vi "Setup Dialog.vi"(0 "State In":T3) -> (4 "State Out":T3, 8 "canceled?":bool)   [LabVIEW 2020, in "KTable.xctl"]
uses:
  KTable.xctl
  State.ctl
  ColumnSpec.ctl
  ColumnType.ctl
  Table Properties.ctl
  Events.ctl
  Event Data.ctl
  Event Type.ctl
  KListbox/KListbox.xctl
  Buttons/KCheckmarkBoolean 2.ctl
panel:
  in  "Show row headers":T1
  in  "Max rows":i32
  in  "User can add/delete rows":T1
  in  "Vertical scrollbar":T1
  out "redisplay":bool
  in  "Tab (top)":enum32{"Page 2"}(tab)
  in  "Name":string
  in  "Type":T2(ring)
  in  "Width":i32
  in  "Position":enum16{"Left", "Center", "Right"}(ring)
  in  "Locked":T1
  in  "Delete Button":bool
  in  "Add Button":bool
  out "cancel signal":bool
  in  "Cancel Button":bool
  in  "OK Button":bool
  in  "Tab (bottom)":T8(tab)
  out "EnumValues":string
  in  "EnumPath":path
  in  "Hide NaN":T1
  in  "False":string
  in  "True":string
  in  "Strings":cluster{"Row":i32, "Items":string[]}(xcontrol)
  in  "Columns":i32(listbox)
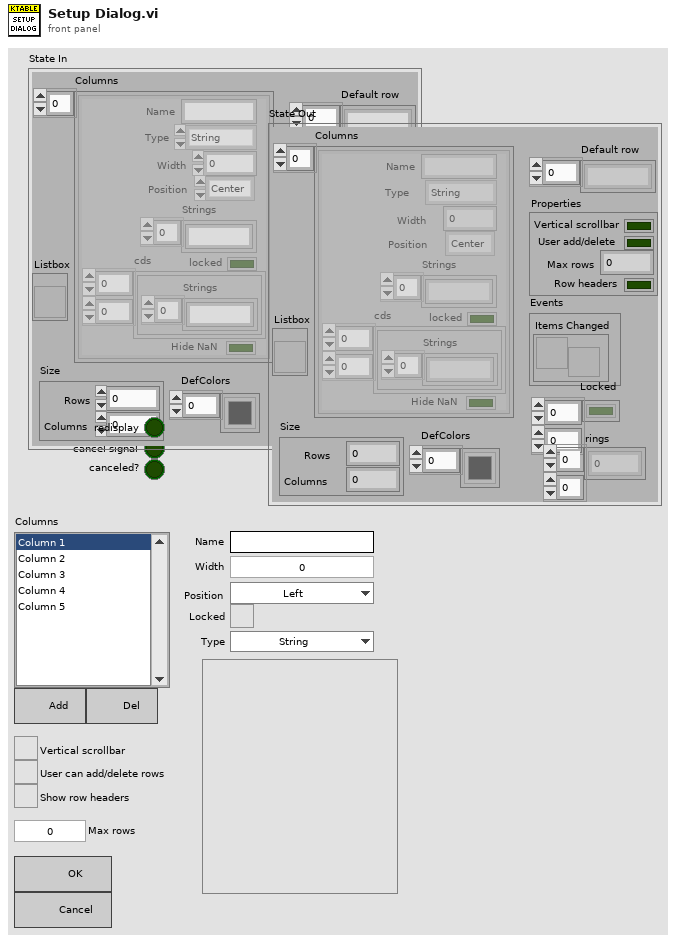
[diagram p1: front panel]
types:
  T1 = typedef "KCheckmarkBoolean 2.ctl" = bool
  T2 = enum16{"String", "Enum", "Int", "Double", "Boolean", "Ring", "Formula", "Color"}
  T3 = typedef "KTable.xctl/State.ctl" = cluster{"Columns":T4[], "Listbox":refnum<vi>, "Default row":string[], "Properties":T6, "Events":T7, "Locked":bool[][], "Size":cluster{"Rows":i32, "Columns":i32}, "rings":i32[][], "DefColors":u32[]}
  T4 = typedef "KTable.xctl/ColumnSpec.ctl" = cluster{"Name":string, "Type":T5, "Width":i32, "Strings":string[], "Position":enum16{"Left", "Center", "Right"}, "locked":bool, "cds":cluster{"Strings":string[]}[][], "Hide NaN":bool}
  T5 = typedef "KTable.xctl/ColumnType.ctl" = enum16{"String", "Enum", "Int", "Double", "Boolean", "Ring", "Formula", "Color"}
  T6 = typedef "KTable.xctl/Table Properties.ctl" = cluster{"Vertical scrollbar":bool, "User add/delete":bool, "Max rows":i32, "Row headers":bool}
  T7 = typedef "KTable.xctl/Events.ctl" = cluster{"Items Changed":refnum<user-event>}
  T8 = enum32{"String", "Enum", "Int", "Double", "Boolean", "Ring", "Formula", "Color"}
  T9 = enum32{"String", "Enum", "Int", "Double", "Boolean", "Ring", "Formula"}
  T10 = enum8{"Enabled", "Disabled", "Disabled and Grayed Out"}
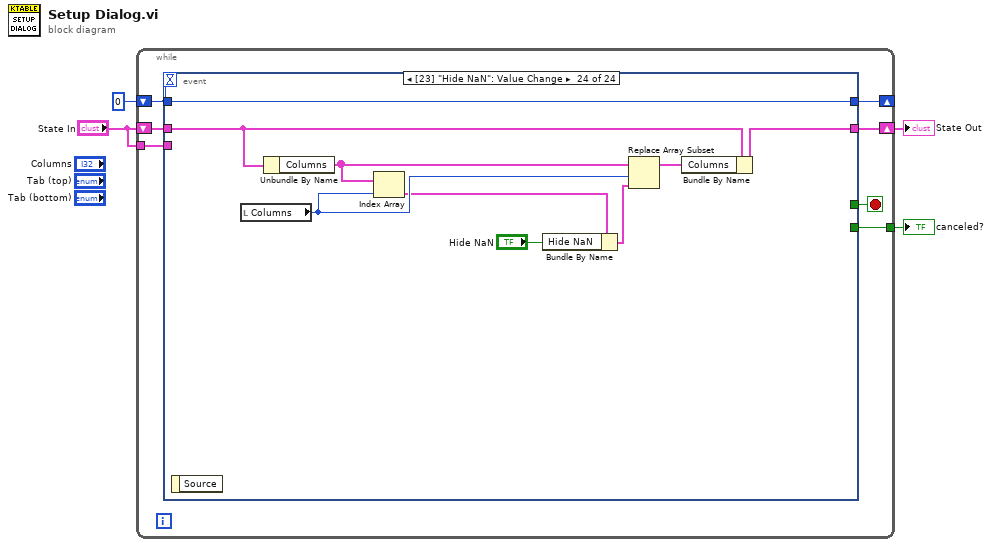
[diagram p0: block diagram]
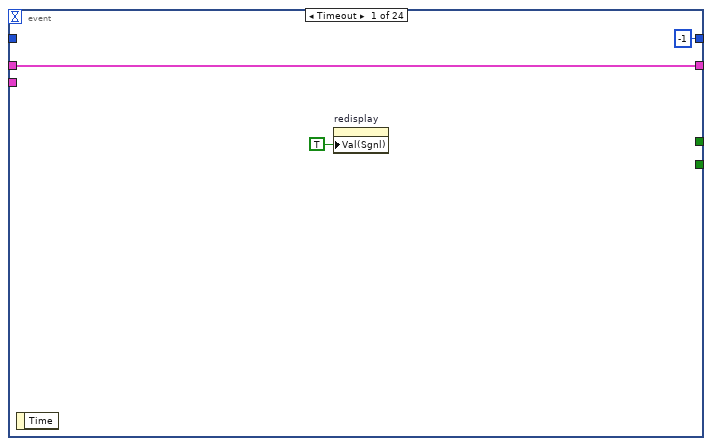
[diagram p2: hidden frame]
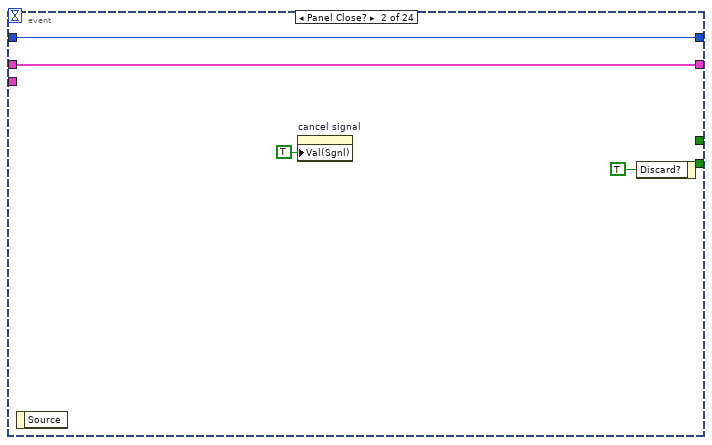
[diagram p3: hidden frame]
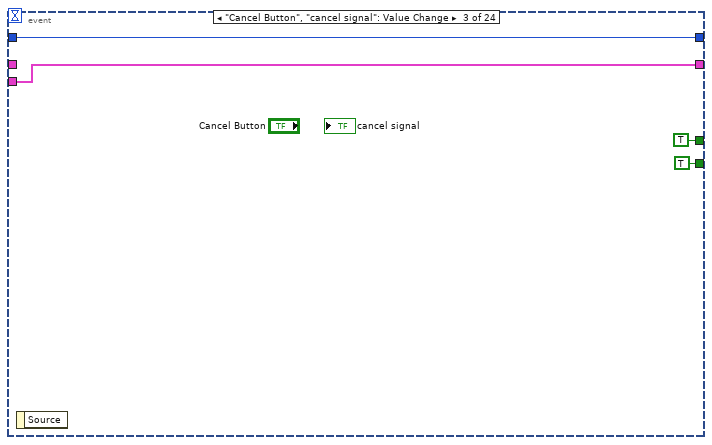
[diagram p4: hidden frame]
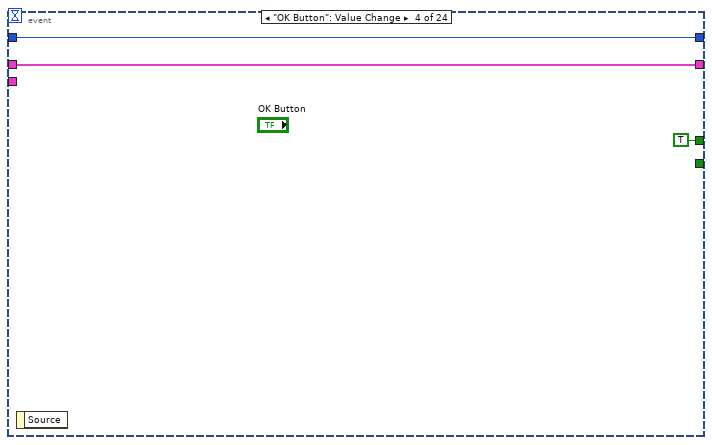
[diagram p5: hidden frame]
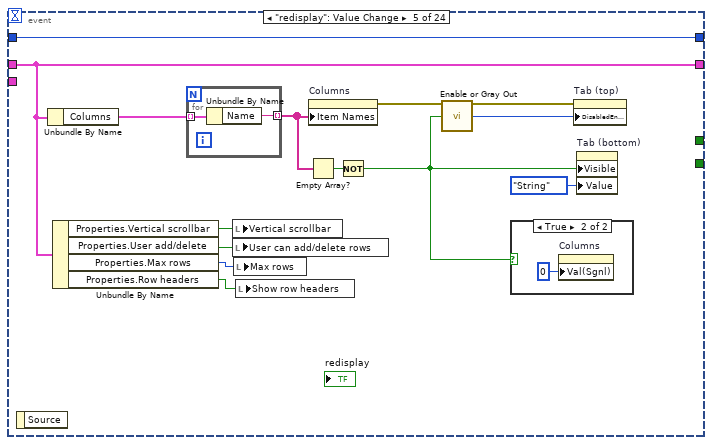
[diagram p6: hidden frame]
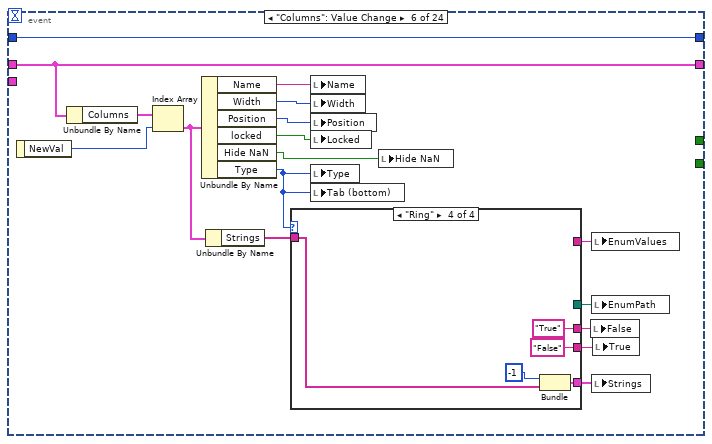
[diagram p8: hidden frame]
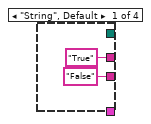
[diagram p9: hidden frame]
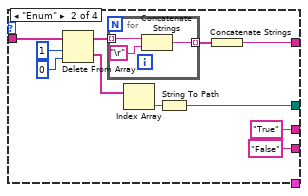
[diagram p10: hidden frame]
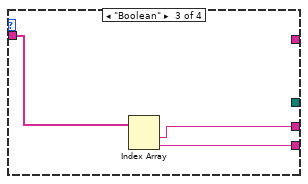
[diagram p11: hidden frame]
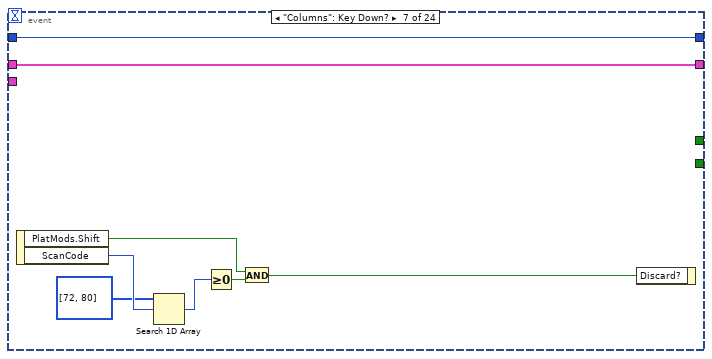
[diagram p12: hidden frame]
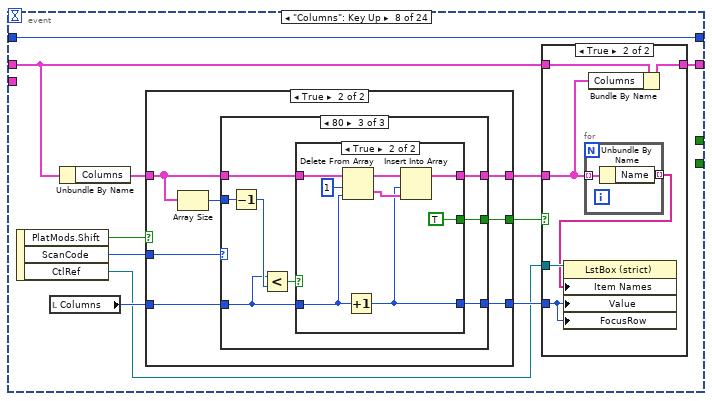
[diagram p13: hidden frame]
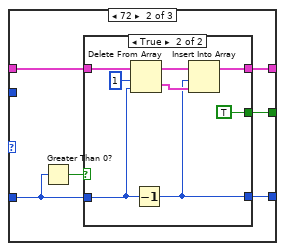
[diagram p17: hidden frame]
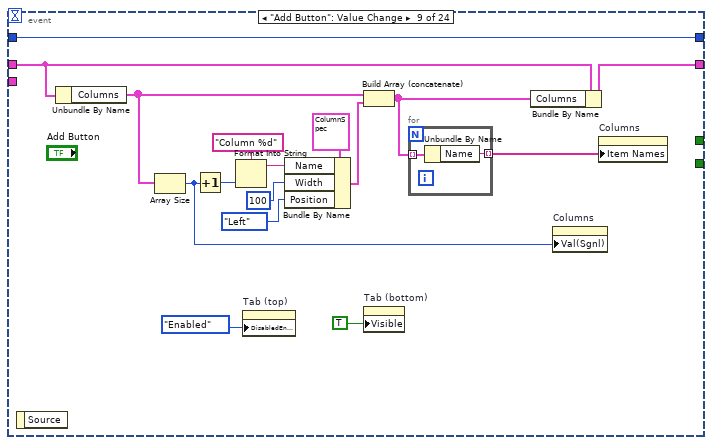
[diagram p20: hidden frame]
diagram:
  n1 = while {
    shift-right: [w10] -> _
    shift-left: 0 -> [w11]
    shift-right: [w7] -> w1
    shift-left: "State In" -> [w8]
    tunnel: "State In" -> [w6]
    tunnel: [w5] -> w2
    stop <- w9 stop-if-true
    n2 = event shown="[23] \"Hide NaN\": Value Change" {
      selector: _ -> [_ _ _ _ _ _ _ _ _ _ _ _ _ _ _ _ _ _ _ _ _ _ _ _]
      dyn-events: _ -> [_ _ _ _ _ _ _ _ _ _ _ _ _ _ _ _ _ _ _ _ _ _ _ _]
      timeout: w11 -> [_ _ _ _ _ _ _ _ _ _ _ _ _ _ _ _ _ _ _ _ _ _ _ _]
      tunnel: w11 -> [_ w18 w22 w25 w31 w58 w90 w101 w171 w180 w190 w194 w198 w202 w212 w225 w234 w243 w256 w274 w289 w301 w311 w320]
      tunnel: [-1 w18 w22 w25 w31 w58 w90 w101 w171 w180 w190 w194 w198 w202 w212 w225 w234 w243 w256 w274 w289 w301 w311 w320] -> w10
      tunnel: [_ _ TRUE TRUE _ _ _ _ _ _ _ _ _ _ _ _ _ _ _ _ _ _ _ _] -> w9
      tunnel: w8 -> [w13 w15 _ w23 w30 w57 w89 w96 w170 w179 w189 w193 w197 w201 w211 w224 w233 w242 w255 w273 w288 w300 w310 w319]
      tunnel: [w13 w15 w20 w23 w30 w57 w89 w95 w164 w176 w188 w192 w196 w200 w205 w219 w228 w237 w251 w268 w285 w297 w307 w316] -> w7
      tunnel: w6 -> [_ _ w20 _ _ _ _ _ _ _ _ _ _ _ _ _ _ _ _ _ _ _ _ _]
      tunnel: [_ _ TRUE _ _ _ _ _ _ _ _ _ _ _ _ _ _ _ _ _ _ _ _ _] -> w5
      event Timeout {
        n3 = event-data() -> ()  [unwired: 1 in, 1 out]
        n4 = property on="redisplay" class="Bool (strict)"("Val(Sgnl)"=TRUE ("Value (Signaling)")) -> ()  [unwired: 2 in, 2 out]
      }
      event Panel Close? {
        n5 = event-data() -> ()  [unwired: 1 in, 1 out]
        n6 = property on="cancel signal" class="Bool (strict)"("Val(Sgnl)"=TRUE ("Value (Signaling)")) -> ()  [unwired: 2 in, 2 out]
        n7 = event-data("Discard?"=TRUE) -> ()  [unwired: 1 in, 1 out]
      }
      event "Cancel Button", "cancel signal": Value Change {
        n8 = event-data() -> ()  [unwired: 1 in, 1 out]
      }
      event "OK Button": Value Change {
        n9 = event-data() -> ()  [unwired: 1 in, 1 out]
      }
      event "redisplay": Value Change {
        n10 = event-data() -> ()  [unwired: 1 in, 1 out]
        n11 = Unbundle By Name(w30) -> ("Columns"=w38:T4[])
        n12 = Unbundle By Name(w30) -> ("Properties.Vertical scrollbar"=w29:bool, "Properties.User add/delete"=w28:bool, "Properties.Max rows"=w27:i32, "Properties.Row headers"=w26:bool)
        n13 = for {
          tunnel: w38 -> [w41] mode=indexing
          tunnel: [w40] -> w37 mode=indexing
          n14 = Unbundle By Name(w41) -> ("Name"=w40:string)
        }
        n15 = local write "Vertical scrollbar"(w29) -> ()
        n16 = local write "User can add/delete rows"(w28) -> ()
        n17 = local write "Max rows"(w27) -> ()
        n18 = local write "Show row headers"(w26) -> ()
        n19 = Empty Array?(array=w37) -> (empty?=w35:bool)
        n20 = property on="Columns" class="LstBox (strict)"("Item Names"=w37) -> (error out=w36:errorcluster)  [unwired: 2 in, 1 out]
        n21 = Not(x=w35) -> (.not. x?=w33:bool)
        n22 = call "Enable or Gray Out.vi"("Boolean"=w33) -> ("Disabled"=w34:T10)
        n23 = case shown="True" w33 {
          frame False {
          }
          frame True {
            n24 = property on="Columns" class="LstBox (strict)"("Val(Sgnl)"=0 ("Value (Signaling)")) -> ()  [unwired: 2 in, 2 out]
          }
        }
        n25 = property on="Tab (top)" class="TabCtl (strict)"(error in=w36, "DisabledEnum"=w34) -> ()  [unwired: 1 in, 2 out]
        n26 = property on="Tab (bottom)" class="TabCtl (strict)"("Visible"=w33, "Value"=T9."String" ("Tab (bottom)")) -> ()  [unwired: 2 in, 2 out]
      }
      event "Columns": Value Change {
        n27 = event-data() -> ("NewVal"=w53:i32)  [unwired: 1 in]
        n28 = Unbundle By Name(w57) -> ("Columns"=w56:T4[])
        n29 = Index Array(array=w56, index=w53) -> (element=w51:T4)
        n30 = Unbundle By Name(w51) -> ("Name"=w55:string, "Width"=w54:i32, "Position"=w52:enum16{"Left", "Center", "Right"}, "locked"=w43:bool, "Hide NaN"=w42:bool, "Type"=w50:T5)
        n31 = Unbundle By Name(w51) -> ("Strings"=w49:string[])
        n32 = case shown="\"Ring\"" w50 {
          tunnel: w49 -> [_ w71 w77 w80]
          tunnel: [_ w67 _ _] -> w48
          tunnel: [_ w65 _ _] -> w47
          tunnel: ["True" ("String") "True" ("String") w76 "True" ("String")] -> w46
          tunnel: ["False" ("String") "False" ("String") w75 "False" ("String")] -> w45
          tunnel: [_ _ _ w78] -> w44
          frame "String", Default {
          }
          frame "Enum" {
            n33 = Delete From Array(array=w71, length=1, index=0) -> (deleted portion=w61:string[], array with subset deleted=w62:string[])
            n34 = for {
              tunnel: w62 -> [w74] mode=indexing
              tunnel: [w72] -> w66 mode=indexing
              n35 = Concatenate Strings(w74, "\r") -> (w72:string)
            }
            n36 = Index Array(array=w61) -> (element=w68:string)  [unwired: 1 in]
            n37 = String To Path(string=w68) -> (path=w67:path)
            n38 = Concatenate Strings(w66) -> (w65:string)
          }
          frame "Boolean" {
            n39 = Index Array(array=w77) -> (element #1=w76:string, element #2=w75:string)  [unwired: 2 in]
          }
          frame "Ring" {
            n40 = Bundle(-1, "Strings"=w80) -> (w78:cluster{i32, "Strings":string[]})  [unwired: 1 in]
          }
        }
        n41 = local write "Name"(w55) -> ()
        n42 = local write "Width"(w54) -> ()
        n43 = local write "Position"(w52) -> ()
        n44 = local write "Locked"(w43) -> ()
        n45 = local write "Type"(w50) -> ()
        n46 = local write "Tab (bottom)"(w50) -> ()
        n47 = local write "Hide NaN"(w42) -> ()
        n48 = local write "False"(w46) -> ()
        n49 = local write "EnumValues"(w47) -> ()
        n50 = local write "EnumPath"(w48) -> ()
        n51 = local write "Strings"(w44) -> ()
        n52 = local write "True"(w45) -> ()
      }
      event "Columns": Key Down? {
        n53 = event-data() -> ("PlatMods.Shift"=w84:bool, "ScanCode"=w88:i16)  [unwired: 1 in]
        n54 = Search 1D Array(1D array=i16[] [72, 80], element=w88) -> (index of element=w86:i32)  [unwired: 1 in]
        n55 = Greater Or Equal To 0?(x=w86) -> (x >= 0?=w85:bool)
        n56 = And(x=w84, y=w85) -> (x .and. y?=w83:bool)
        n57 = event-data("Discard?"=w83) -> ()  [unwired: 1 in, 1 out]
      }
      event "Columns": Key Up {
        n58 = event-data() -> ("PlatMods.Shift"=w100:bool, "ScanCode"=w99:i16, "CtlRef"=w91:refnum<vi>)  [unwired: 1 in]
        n59 = local read "Columns"() -> (w97:i32)
        n60 = Unbundle By Name(w96) -> ("Columns"=w98:T4[])
        n61 = case shown="True" w100 {
          tunnel: w99 -> [_ w119]
          tunnel: w98 -> [w111 w118]
          tunnel: w97 -> [w112 w116]
          tunnel: [w112 w115] -> w92
          tunnel: [w111 w114] -> w94
          tunnel: [_ w113] -> w93
          frame False {
          }
          frame True {
            n62 = Array Size(array=w118) -> (size(s)=w117:i32)
            n63 = case shown="80" w119 {
              tunnel: w118 -> [w121 w126 w145]
              tunnel: w117 -> [_ _ w140]
              tunnel: w116 -> [w120 w125 w138]
              tunnel: [w120 w124 w144] -> w115
              tunnel: [w121 w123 w143] -> w114
              tunnel: [_ w122 w142] -> w113
              frame 0, Default {
              }
              frame 72 {
                n64 = Greater Than 0?(x=w125) -> (x > 0?=w127:bool)
                n65 = case shown="True" w127 {
                  tunnel: w126 -> [w128 w137]
                  tunnel: w125 -> [w129 w133]
                  tunnel: [w129 w132] -> w124
                  tunnel: [w128 w131] -> w123
                  tunnel: [_ TRUE] -> w122
                  frame False {
                  }
                  frame True {
                    n66 = Delete From Array(array=w137, length=1, index=w133) -> (deleted portion=w134:T4[], array with subset deleted=w135:T4[])
                    n67 = Decrement(x=w133) -> (x-1=w132:i32)
                    n68 = Insert Into Array(array=w135, index=w132, new element=w134) -> (w131:T4[])
                  }
                }
              }
              frame 80 {
                n69 = Decrement(x=w140) -> (x-1=w139:i32)
                n70 = Less?(x=w138, y=w139) -> (x < y?=w141:bool)
                n71 = case shown="True" w141 {
                  tunnel: w145 -> [w146 w155]
                  tunnel: w138 -> [w147 w151]
                  tunnel: [w147 w150] -> w144
                  tunnel: [w146 w149] -> w143
                  tunnel: [_ TRUE] -> w142
                  frame False {
                  }
                  frame True {
                    n72 = Delete From Array(array=w155, length=1, index=w151) -> (deleted portion=w152:T4[], array with subset deleted=w153:T4[])
                    n73 = Increment(x=w151) -> (x+1=w150:i32)
                    n74 = Insert Into Array(array=w153, index=w150, new element=w152) -> (w149:T4[])
                  }
                }
              }
            }
          }
        }
        n75 = case shown="True" w93 {
          tunnel: w96 -> [w102 w108]
          tunnel: [w102 w107] -> w95
          tunnel: w94 -> [_ w105]
          tunnel: w92 -> [_ w103]
          tunnel: w91 -> [_ w106]
          frame False {
          }
          frame True {
            n76 = for {
              tunnel: w105 -> [w110] mode=indexing
              tunnel: [w109] -> w104 mode=indexing
              n77 = Unbundle By Name(w110) -> ("Name"=w109:string)
            }
            n78 = property class="LstBox (strict)"(reference=w106, "Item Names"=w104, "Value"=w103, "FocusRow"=w103) -> ()  [unwired: 1 in, 2 out]
            n79 = Bundle By Name(cluster=w108, "Columns"=w105) -> (w107:T3)
          }
        }
      }
      event "Add Button": Value Change {
        n80 = event-data() -> ()  [unwired: 1 in, 1 out]
        n81 = Unbundle By Name(w170) -> ("Columns"=w163:T4[])
        n82 = Array Size(array=w163) -> (size(s)=w158:i32)
        n83 = Increment(x=w158) -> (x+1=w157:i32)
        n84 = Format Into String(format string="Column %d", w157) -> (resulting string=w167:string)  [unwired: 2 in, 1 out]
        n85 = property on="Tab (top)" class="TabCtl (strict)"("DisabledEnum"=T10."Enabled" ("Disabled")) -> ()  [unwired: 2 in, 2 out]
        n86 = Bundle By Name(cluster=T4 {"Name"="", "Type"=enum."String", "Width"=0, "Strings"=[], "Position"=enum."Left", "locked"=FALSE, "cds"=[], "Hide NaN"=FALSE} ("ColSpec"), "Name"=w167, "Width"=100, "Position"=enum16{"Left", "Center", "Right"}."Left") -> (w165:T4)
        n87 = Build Array (concatenate)(w163, w165) -> (w160:T4[])
        n88 = property on="Tab (bottom)" class="TabCtl (strict)"("Visible"=TRUE) -> ()  [unwired: 2 in, 2 out]
        n89 = for {
          tunnel: w160 -> [w173] mode=indexing
          tunnel: [w172] -> w159 mode=indexing
          n90 = Unbundle By Name(w173) -> ("Name"=w172:string)
        }
        n91 = Bundle By Name(cluster=w170, "Columns"=w160) -> (w164:T3)
        n92 = property on="Columns" class="LstBox (strict)"("Val(Sgnl)"=w158) -> ()  [unwired: 2 in, 2 out]
        n93 = property on="Columns" class="LstBox (strict)"("Item Names"=w159) -> ()  [unwired: 2 in, 2 out]
      }
      event "Delete Button": Value Change {
        n94 = event-data() -> ()  [unwired: 1 in, 1 out]
        n95 = Unbundle By Name(w179) -> ("Columns"=w177:T4[])
        n96 = local read "Columns"() -> (w174:i32)
        n97 = Empty Array?(array=w177) -> (empty?=w178:bool)
        n98 = case shown="False" w178 {
          tunnel: w177 -> [w185 w186]
          tunnel: [w184 w186] -> w175
          tunnel: w174 -> [w182 _]
          frame False {
            n99 = Delete From Array(array=w185, length=1, index=w182) -> (array with subset deleted=w184:T4[])  [unwired: 1 out]
            n100 = property on="redisplay" class="Bool (strict)"("Val(Sgnl)"=TRUE ("Value (Signaling)")) -> ()  [unwired: 2 in, 2 out]
          }
          frame True {
          }
        }
        n101 = Bundle By Name(cluster=w179, "Columns"=w175) -> (w176:T3)
      }
      event Value Change {
        n102 = event-data() -> ()  [unwired: 1 in, 1 out]
        n103 = Bundle By Name(cluster=w189, "Properties.Vertical scrollbar"="Vertical scrollbar") -> (w188:T3)
      }
      event Value Change {
        n104 = event-data() -> ()  [unwired: 1 in, 1 out]
        n105 = Bundle By Name(cluster=w193, "Properties.User add/delete"="User can add/delete rows") -> (w192:T3)
      }
      event Value Change {
        n106 = event-data() -> ()  [unwired: 1 in, 1 out]
        n107 = Bundle By Name(cluster=w197, "Properties.Row headers"="Show row headers") -> (w196:T3)
      }
      event "Max rows": Value Change {
        n108 = event-data() -> ()  [unwired: 1 in, 1 out]
        n109 = Bundle By Name(cluster=w201, "Properties.Max rows"="Max rows") -> (w200:T3)
      }
      event "Name": Value Change {
        n110 = event-data() -> ()  [unwired: 1 in, 1 out]
        n111 = local read "Columns"() -> (w207:i32)
        n112 = Unbundle By Name(w211) -> ("Columns"=w208:T4[])
        n113 = Index Array(array=w208, index=w207) -> (element=w210:T4)
        n114 = Bundle By Name(cluster=w210, "Name"="Name") -> (w206:T4)
        n115 = Replace Array Subset(array=w208, new element=w206, index=w207) -> (w203:T4[])
        n116 = Bundle By Name(cluster=w211, "Columns"=w203) -> (w205:T3)
        n117 = for {
          tunnel: w203 -> [w214] mode=indexing
          tunnel: [w213] -> w204 mode=indexing
          n118 = Unbundle By Name(w214) -> ("Name"=w213:string)
        }
        n119 = property on="Columns" class="LstBox (strict)"("Item Names"=w204) -> ()  [unwired: 2 in, 2 out]
      }
      event "Width": Value Change {
        n120 = event-data() -> ()  [unwired: 1 in, 1 out]
        n121 = local read "Columns"() -> (w221:i32)
        n122 = Unbundle By Name(w224) -> ("Columns"=w222:T4[])
        n123 = Max & Min(x="Width", y=10) -> (max(x,y)=w215:i32)  [unwired: 1 out]
        n124 = Index Array(array=w222, index=w221) -> (element=w223:T4)
        n125 = Bundle By Name(cluster=w223, "Width"=w215) -> (w220:T4)
        n126 = local write "Width"(w215) -> ()
        n127 = Replace Array Subset(array=w222, new element=w220, index=w221) -> (w218:T4[])
        n128 = Bundle By Name(cluster=w224, "Columns"=w218) -> (w219:T3)
      }
      event "Position": Value Change {
        n129 = event-data() -> ()  [unwired: 1 in, 1 out]
        n130 = local read "Columns"() -> (w230:i32)
        n131 = Unbundle By Name(w233) -> ("Columns"=w231:T4[])
        n132 = Index Array(array=w231, index=w230) -> (element=w232:T4)
        n133 = Bundle By Name(cluster=w232, "Position"="Position") -> (w229:T4)
        n134 = Replace Array Subset(array=w231, new element=w229, index=w230) -> (w227:T4[])
        n135 = Bundle By Name(cluster=w233, "Columns"=w227) -> (w228:T3)
      }
      event Value Change {
        n136 = event-data() -> ()  [unwired: 1 in, 1 out]
        n137 = local read "Columns"() -> (w239:i32)
        n138 = Unbundle By Name(w242) -> ("Columns"=w240:T4[])
        n139 = Index Array(array=w240, index=w239) -> (element=w241:T4)
        n140 = Bundle By Name(cluster=w241, "locked"="Locked") -> (w238:T4)
        n141 = Replace Array Subset(array=w240, new element=w238, index=w239) -> (w236:T4[])
        n142 = Bundle By Name(cluster=w242, "Columns"=w236) -> (w237:T3)
      }
      event "Type": Value Change {
        n143 = event-data() -> ()  [unwired: 1 in, 1 out]
        n144 = local read "Columns"() -> (w252:i32)
        n145 = local read "False"() -> (w246:string)
        n146 = local read "True"() -> (w245:string)
        n147 = Unbundle By Name(w255) -> ("Columns"=w253:T4[])
        n148 = Build Array(w246, w245) -> (w244:string[])
        n149 = Index Array(array=w253, index=w252) -> (element=w254:T4)
        n150 = Bundle By Name(cluster=w254, "Type"="Type") -> (w247:T4)
        n151 = local write "Tab (bottom)"("Type") -> ()
        n152 = case shown="\"Boolean\"" "Type" {
          tunnel: [w257 w259] -> w248
          tunnel: w247 -> [w257 w260]
          tunnel: w244 -> [_ w258]
          frame "String", Default {
          }
          frame "Boolean" {
            n153 = Bundle By Name(cluster=w260, "Strings"=w258) -> (w259:T4)
          }
        }
        n154 = Replace Array Subset(array=w253, new element=w248, index=w252) -> (w250:T4[])
        n155 = Bundle By Name(cluster=w255, "Columns"=w250) -> (w251:T3)
      }
      event "EnumPath": Value Change {
        n156 = event-data() -> ()  [unwired: 1 in, 1 out]
        n157 = local read "Columns"() -> (w270:i32)
        n158 = Unbundle By Name(w273) -> ("Columns"=w271:T4[])
        n159 = call "Get Enum Strings From File.vi"("EnumPath"="EnumPath") -> ("Strings []"=w266:string[])  [unwired: 9 in, 1 out]
        n160 = Path To String(path="EnumPath") -> (string=w262:string)
        n161 = Build Array (concatenate)(w262, w266) -> (w263:string[])
        n162 = Index Array(array=w271, index=w270) -> (element=w272:T4)
        n163 = for {
          tunnel: w266 -> [w277] mode=indexing
          tunnel: [w275] -> w265 mode=indexing
          n164 = Concatenate Strings(w277, "\r") -> (w275:string)
        }
        n165 = Bundle By Name(cluster=w272, "Strings"=w263) -> (w269:T4)
        n166 = Replace Array Subset(array=w271, new element=w269, index=w270) -> (w267:T4[])
        n167 = Concatenate Strings(w265) -> (→"EnumValues":string)
        n168 = Bundle By Name(cluster=w273, "Columns"=w267) -> (w268:T3)
      }
      event "True": Value Change {
        n169 = event-data() -> ()  [unwired: 1 in, 1 out]
        n170 = local read "Columns"() -> (w286:i32)
        n171 = Unbundle By Name(w288) -> ("Columns"=w287:T4[])
        n172 = Index Array(array=w287, index=w286) -> (element=w281:T4)
        n173 = Unbundle By Name(w281) -> ("Strings"=w283:string[])
        n174 = Replace Array Subset(array=w283, new element="True", index=1) -> (w280:string[])
        n175 = Bundle By Name(cluster=w281, "Strings"=w280) -> (w279:T4)
        n176 = Replace Array Subset(array=w287, new element=w279, index=w286) -> (w284:T4[])
        n177 = Bundle By Name(cluster=w288, "Columns"=w284) -> (w285:T3)
      }
      event "False": Value Change {
        n178 = event-data() -> ()  [unwired: 1 in, 1 out]
        n179 = local read "Columns"() -> (w298:i32)
        n180 = Unbundle By Name(w300) -> ("Columns"=w299:T4[])
        n181 = Index Array(array=w299, index=w298) -> (element=w293:T4)
        n182 = Unbundle By Name(w293) -> ("Strings"=w295:string[])
        n183 = Replace Array Subset(array=w295, new element="False", index=0) -> (w292:string[])
        n184 = Bundle By Name(cluster=w293, "Strings"=w292) -> (w291:T4)
        n185 = Replace Array Subset(array=w299, new element=w291, index=w298) -> (w296:T4[])
        n186 = Bundle By Name(cluster=w300, "Columns"=w296) -> (w297:T3)
      }
      event "Strings": Value Change {
        n187 = event-data() -> ()  [unwired: 1 in, 1 out]
        n188 = local read "Columns"() -> (w308:i32)
        n189 = Unbundle By Name(w310) -> ("Columns"=w309:T4[])
        n190 = Index Array(array=w309, index=w308) -> (element=w305:T4)
        n191 = Unbundle By Name("Strings") -> ("Items"=w302:string[])
        n192 = Bundle By Name(cluster=w305, "Strings"=w302) -> (w304:T4)
        n193 = Replace Array Subset(array=w309, new element=w304, index=w308) -> (w306:T4[])
        n194 = Bundle By Name(cluster=w310, "Columns"=w306) -> (w307:T3)
      }
      event Value Change {
        n195 = event-data() -> ()  [unwired: 1 in, 1 out]
        n196 = local read "Columns"() -> (w317:i32)
        n197 = Unbundle By Name(w319) -> ("Columns"=w318:T4[])
        n198 = Index Array(array=w318, index=w317) -> (element=w314:T4)
        n199 = Bundle By Name(cluster=w314, "Hide NaN"="Hide NaN") -> (w313:T4)
        n200 = Replace Array Subset(array=w318, new element=w313, index=w317) -> (w315:T4[])
        n201 = Bundle By Name(cluster=w319, "Columns"=w315) -> (w316:T3)
      }
    }
  }
  "State Out" <- w1
  "canceled?" <- w2
